vi "close.vi"(8 "error in (no error)":errorcluster, 11 "LibReader in":refnum<class "LibReader.lvclass">) -> (0 "error out":errorcluster, 3 "LibReader out":refnum<class "LibReader.lvclass">)   [LabVIEW 2018, in "LibReader.lvclass"]
doc: "Close the internal references."
uses:
  LibReader.lvclass
  LibReader.lvclass/LibReader.ctl
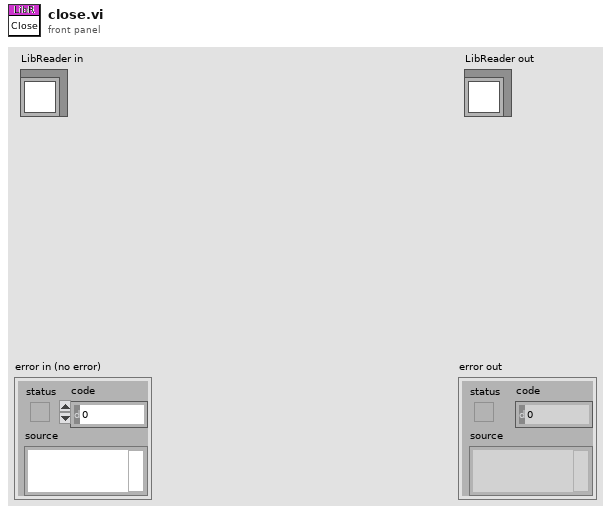
[diagram p1: front panel]
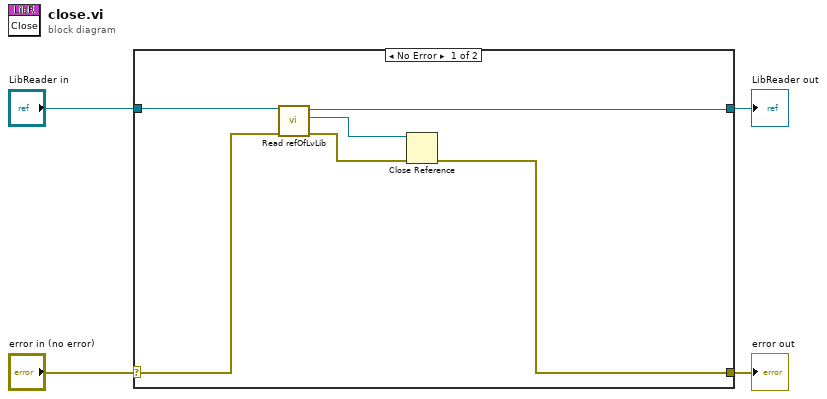
[diagram p0: block diagram]
diagram:
  n1 = case shown="No Error" "error in (no error)" {
    selector: "error in (no error)" -> [w8 w12]
    tunnel: [w5 w12] -> w3
    tunnel: [w9 w11] -> w1
    tunnel: "LibReader in" -> [w10 w11]
    frame No Error {
      n2 = call "Read refOfLvLib.vi"("error in (no error)"=w8, "LibReader in"=w10) -> ("error out"=w6:errorcluster, "refOfLvLib"=w7:refnum<vi>, "LibReader out"=w9:refnum<class "LibReader.lvclass">)  [unwired: 7 in]
      n3 = Close Reference(reference=w7, error in (no error)=w6) -> (error out=w5:errorcluster)
    }
    frame Error {
    }
  }
  "error out" <- w3
  "LibReader out" <- w1
